vi "HemisphereFlashingTest.vi"() -> ()   [LabVIEW 2013]
uses:
  <vilib>/Instr/_visa.llb/VISA Configure Serial Port (Instr).vi
panel:
  out "error out":errorcluster
  out "read buffer":string
  in  "Input\nbuffer size":u32=4096
  in  "error in (no error)":errorcluster
  in  "VISA Refnum in":refnum<visa-resource-name>
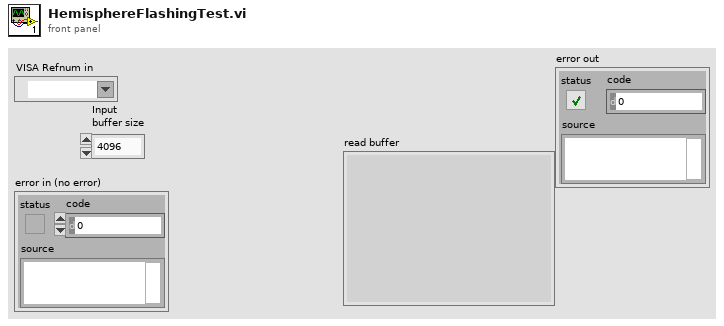
[diagram p1: front panel]
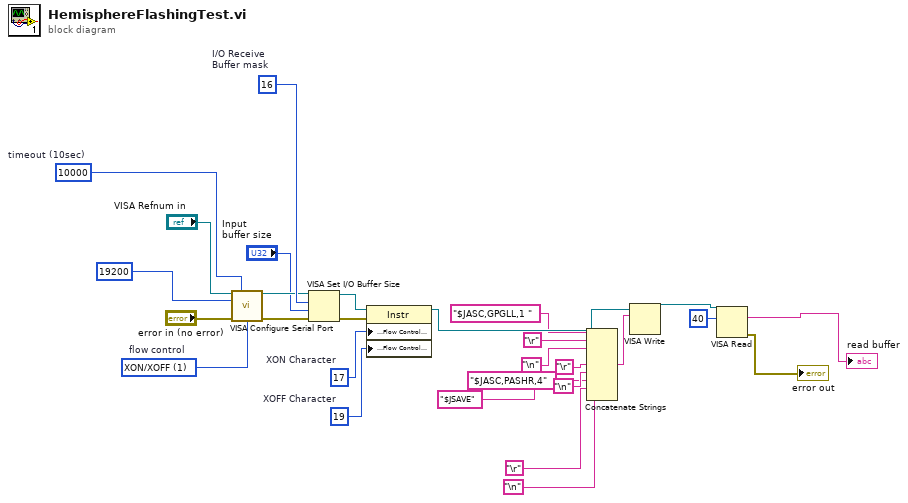
[diagram p0: block diagram]
diagram:
  w25 = u32 10000  # timeout (10sec)
  w22 = u8 19  # XOFF Character
  w21 = u8 17  # XON Character
  w26 = u16 16  # I/O Receive Buffer mask
  w17 = u16 1 items=["None"=0, "XON/XOFF"=1, "RTS/CTS"=2, "DTR/DSR"=4]  # flow control
  n1 = call-poly "VISA Configure Serial Port"("VISA resource name"="VISA Refnum in", "timeout (10sec)"=w25, "baud rate (9600)"=u32 19200, "error in (no error)"="error in (no error)", "flow control (0:none)"=w17) -> ("VISA resource name out"=w23:refnum<visa-resource-name>, "error out"=w24:errorcluster)  [unwired: 9 in]
  n2 = VISA Set I/O Buffer Size(VISA resource name=w23, mask (16)=w26, size (4096)="Input\nbuffer size", error in (no error)=w24) -> (VISA resource name out=w19:refnum<visa-resource-name>, error out=w20:errorcluster)
  n3 = property class="Instr"(reference=w19, error in=w20, "Serial Settings:Flow Control XON Character"=w21, "Serial Settings:Flow Control XOFF Character"=w22) -> (reference out=w15:refnum<visa-resource-name>)  [unwired: 1 out]
  n4 = Concatenate Strings("$JASC,GPGLL,1 " ("write buffer"), "\r", "\n", "$JASC,PASHR,4" ("string"), "\r", "\n", "$JSAVE" ("string"), "\r", "\n") -> (w10:string)
  n5 = VISA Write(VISA resource name=w15, write buffer=w10) -> (VISA resource name out=w12:refnum<visa-resource-name>)  [unwired: 1 in, 2 out]
  n6 = VISA Read(VISA resource name=w12, byte count=u32 40) -> (read buffer=→"read buffer":string, error out=→"error out":errorcluster)  [unwired: 1 in, 2 out]
